vi "菜单-保存.vi"(8 "error in (no error)":errorcluster caption="错误输入（无错误）", 11 "程序响应 输入":refnum<class "程序响应.lvclass">) -> (0 "error out":errorcluster caption="错误输出", 3 "程序响应 输出":refnum<class "程序响应.lvclass">)   [LabVIEW 2020, in "程序响应.lvlib" / "程序响应.lvclass"]
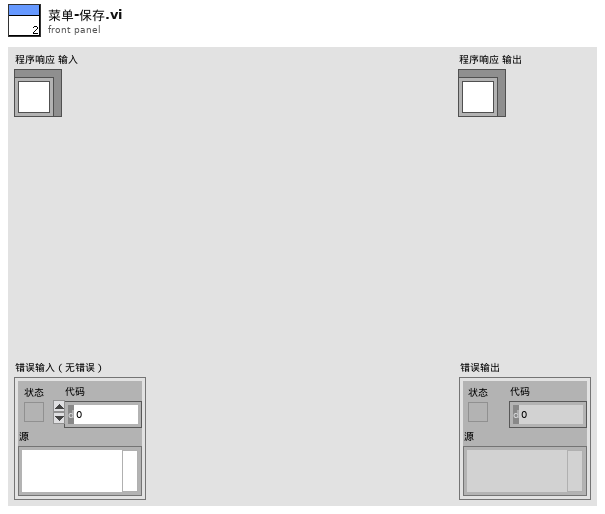
[diagram p1: front panel]
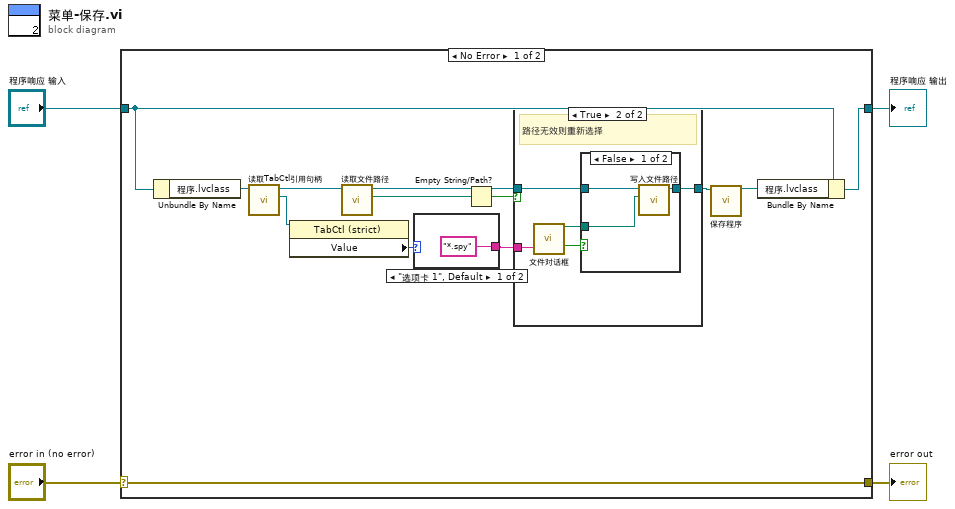
[diagram p0: block diagram]
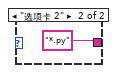
[diagram p2: hidden frame]
diagram:
  n1 = case shown="No Error" "error in (no error)" {
    selector: "error in (no error)" -> [w17 w31]
    tunnel: [w17 w31] -> w3
    tunnel: [w13 w30] -> w1
    tunnel: "程序响应 输入" -> [w14 w30]
    frame No Error {
      n2 = Unbundle By Name(w14) -> ("程序.lvclass"=w7:refnum<class "程序.lvclass">)
      n3 = call-dynamic "读取TabCtl引用句柄.vi"("程序输入"=w7) -> ("TabCtl引用句柄"=w9:refnum<vi>, "程序输出"=w5:refnum<class "程序.lvclass">)  [unwired: 8 in, 1 out]
      n4 = property class="TabCtl (strict)"(reference=w9) -> ("Value"=w8:enum32{"选项卡 1", "选项卡 2"})  [unwired: 1 in, 2 out]
      n5 = call-dynamic "读取文件路径.vi"("程序输入"=w5) -> ("文件路径"=w12:path, "程序输出"=w11:refnum<class "程序.lvclass">)  [unwired: 8 in, 1 out]
      n6 = case shown="\"选项卡 1\", Default" w8 {
        tunnel: ["*.spy" ("pattern (all files)") "*.py" ("pattern (all files)")] -> w6
        frame "选项卡 1", Default {
        }
        frame "选项卡 2" {
        }
      }
      n7 = Empty String/Path?(string/path=w12) -> (empty?=w16:bool)
      n8 = case shown="True" w16 {
        tunnel: w11 -> [w20 w25]
        tunnel: [w20 w24] -> w10
        tunnel: w6 -> [_ w21]
        frame False {
          # "路径有效则直接保存"
        }
        frame True {
          # "路径无效则重新选择"
          n9 = call "文件对话框"("pattern (all files)"=w21) -> ("selected path"=w23:path, "cancelled"=w22:bool)  [unwired: 11 in, 2 out]
          n10 = case shown="False" w22 {
            tunnel: w25 -> [w28 w29]
            tunnel: [w27 w29] -> w24
            tunnel: w23 -> [w26 _]
            frame False {
              n11 = call-dynamic "写入文件路径.vi"("文件路径"=w26, "程序输入"=w28) -> ("程序输出"=w27:refnum<class "程序.lvclass">)  [unwired: 8 in, 1 out]
            }
            frame True {
            }
          }
        }
      }
      n12 = call-dynamic "保存程序.vi"("程序 输入"=w10) -> ("程序 输出"=w15:refnum<class "程序.lvclass">)  [unwired: 9 in, 1 out]
      n13 = Bundle By Name(cluster=w14, "程序.lvclass"=w15) -> (w13:refnum<class "程序响应.lvclass">)
    }
    frame Error {
    }
  }
  "error out" <- w3
  "程序响应 输出" <- w1
